vi "Gare ratio save FGV.vi"(7 "Command":T1(ring), 8 "error in (no error)":errorcluster, 10 "Gear Ratio":dbl=4.3, 11 "File Path":path) -> (0 "error out":errorcluster, 2 "Gear Ratio":dbl=4.3)   [LabVIEW 2018]
doc: "This Subvi usde for CSV Initialize ,Read, Write and close.\nIntilise case; we check File avaliblity in not found create csv file\nRead Case ; Read data from csv file"
uses:
  <vilib>/Utility/file.llb/Write Delimited Spreadsheet (string).vi
  <vilib>/Utility/file.llb/Read Delimited Spreadsheet (string).vi
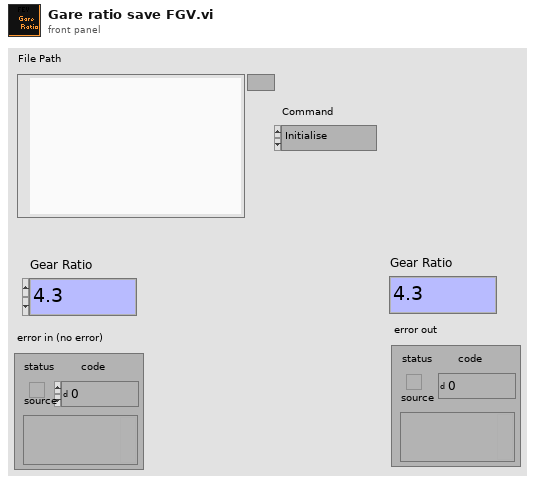
[diagram p1: front panel]
types:
  T1 = enum16{"Initialise", "Read Data", "Write Data", "Close"}
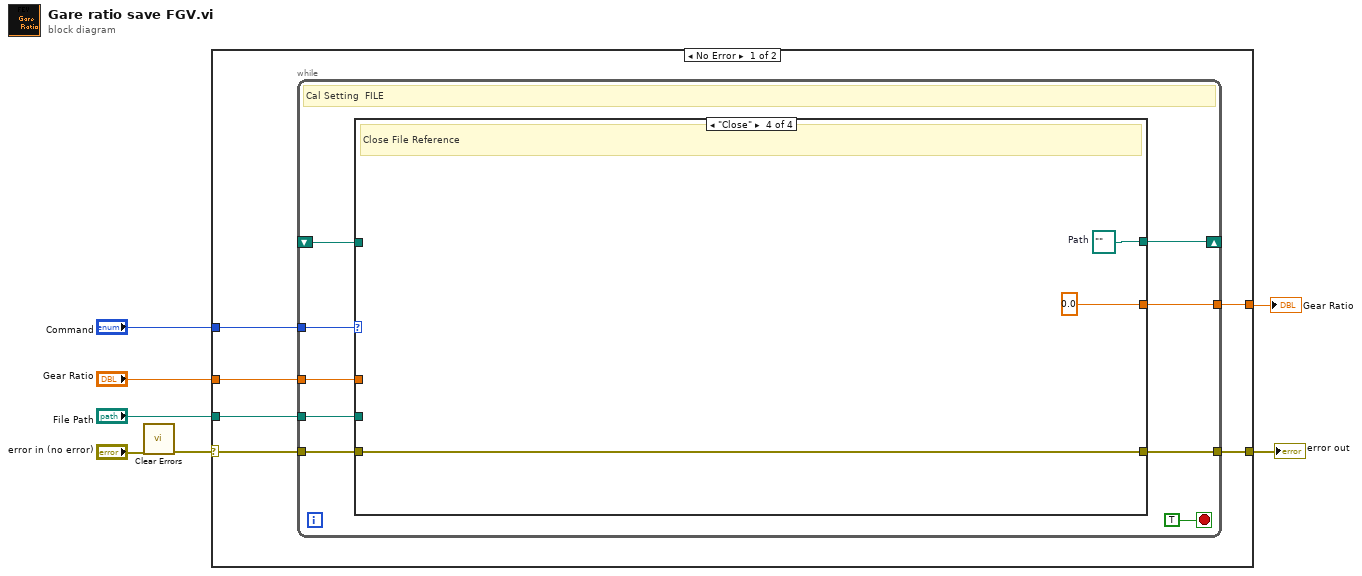
[diagram p0: block diagram]
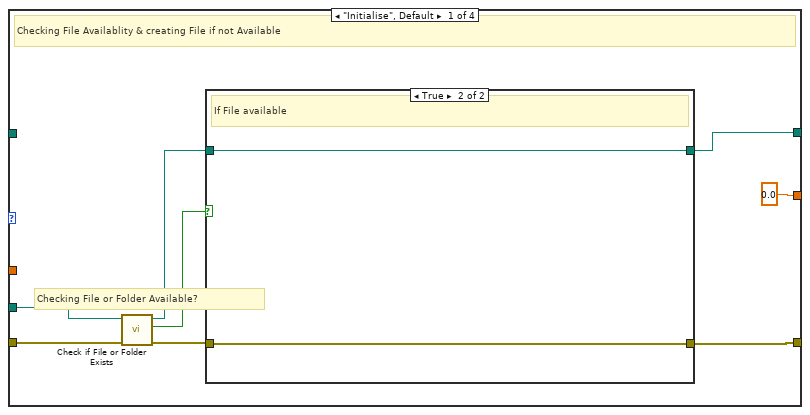
[diagram p2: hidden frame]
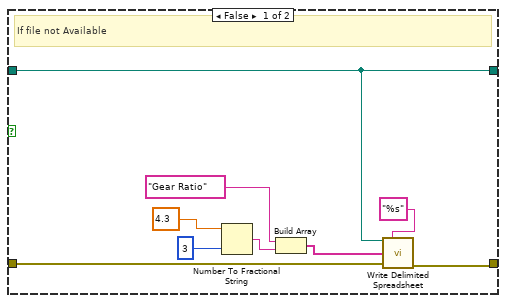
[diagram p3: hidden frame]
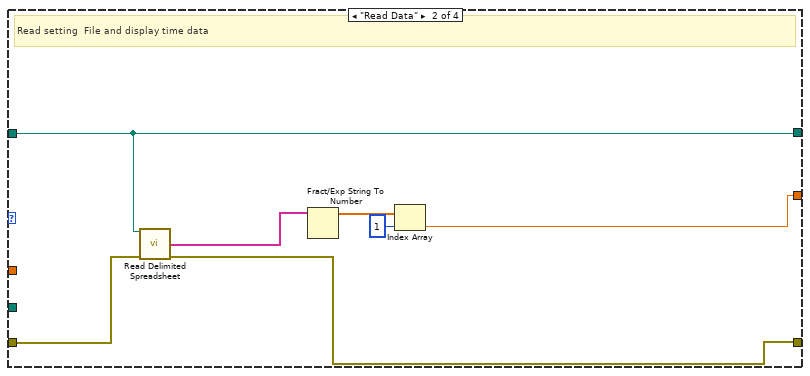
[diagram p4: hidden frame]
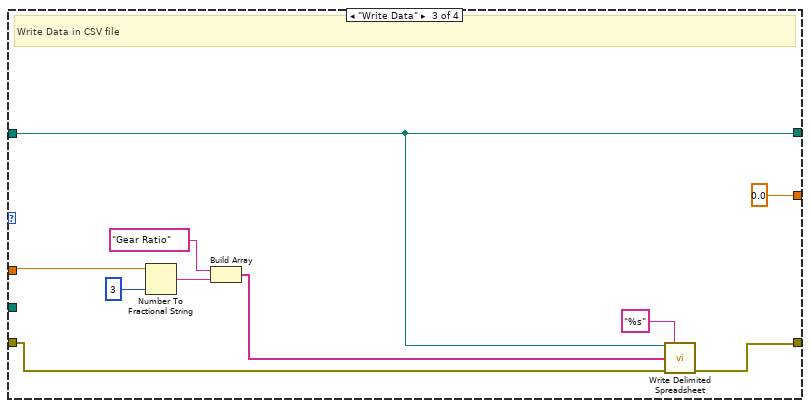
[diagram p5: hidden frame]
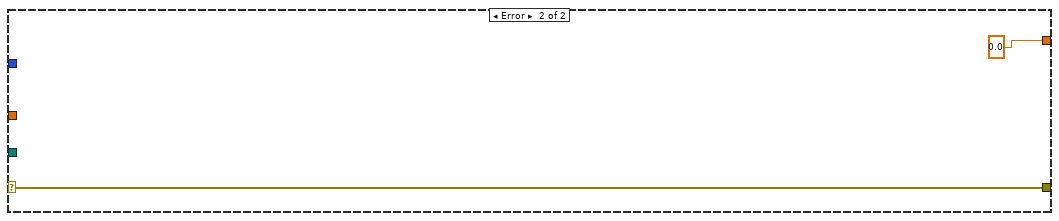
[diagram p6: hidden frame]
diagram:
  n1 = call <vilib>:"Clear Errors.vi"("error in (no error)"="error in (no error)") -> ("error out"=w3:errorcluster)  [unwired: 5 in, 1 out]
  n2 = case shown="No Error" w3 {
    selector: w3 -> [w12 w63]
    tunnel: [w11 w63] -> w6
    tunnel: "Command" -> [w13 _]
    tunnel: "File Path" -> [w10 _]
    tunnel: [w9 0.0 ("Gear Ratio")] -> w2
    tunnel: "Gear Ratio" -> [w8 _]
    frame No Error {
      n3 = while {
        shift-right: [w17] -> _
        shift-left: _ -> [w16]
        tunnel: w13 -> [w21]
        tunnel: w12 -> [w20]
        tunnel: [w19] -> w11
        tunnel: w10 -> [w18]
        tunnel: [w15] -> w9
        tunnel: w8 -> [w14]
        stop <- TRUE stop-if-true
        # "Cal Setting  FILE"
        n4 = case shown="\"Close\"" w21 {
          tunnel: w20 -> [w30 w47 w55 w61]
          tunnel: [w24 w46 w54 w61] -> w19
          tunnel: w18 -> [w29 _ _ _]
          tunnel: [w27 w48 w53 w60] -> w17
          tunnel: w16 -> [_ w48 w53 _]
          tunnel: [0.0 ("Gear Ratio") w43 0.0 ("Gear Ratio") 0.0 ("Gear Ratio")] -> w15
          tunnel: w14 -> [_ _ w51 _]
          frame "Initialise", Default {
            # "Checking File or Folder Available?"
            # "Checking File Availablity & creating File if not Available"
            n5 = call <vilib>:"Check if File or Folder Exists.vi"("error in (no error)"=w30, "path"=w29) -> ("error out"=w25:errorcluster, "file or folder exists?"=w28:bool, "dup path"=w26:path)  [unwired: 7 in]
            n6 = case shown="True" w28 {
              tunnel: [w37 w41] -> w27
              tunnel: w26 -> [w37 w41]
              tunnel: w25 -> [w35 w40]
              tunnel: [w34 w40] -> w24
              frame False {
                # "If file not Available"
                n7 = Number To Fractional String(number=4.3, precision (6)=i16 3) -> (F-format string=w39:string)  [unwired: 2 in]
                n8 = Build Array("Gear Ratio" ("Output Load Offset (Kg)"), w39) -> (w31:string[])
                n9 = call-poly <vilib>:"Write Delimited Spreadsheet.vi"("file path (dialog if empty)"=w37, "format (%s)"="%s", "1D data"=w31, "error in (no error)"=w35) -> ("error out"=w34:errorcluster)  [unwired: 10 in, 1 out]
              }
              frame True {
                # "If File available"
              }
            }
          }
          frame "Read Data" {
            # "Read setting  File and display time data"
            n10 = call-poly <vilib>:"Read Delimited Spreadsheet.vi"("file path (dialog if empty)"=w48, "error in (no error)"=w47) -> ("first row"=w44:string[], "error out"=w46:errorcluster)  [unwired: 8 in, 4 out]
            n11 = Fract/Exp String To Number(string=w44) -> (number=w45:dbl[])  [unwired: 3 in, 1 out]
            n12 = Index Array(array=w45, index=1) -> (element=w43:dbl)
          }
          frame "Write Data" {
            # "Write Data in CSV file"
            n13 = Number To Fractional String(number=w51, precision (6)=i16 3) -> (F-format string=w58:string)  [unwired: 2 in]
            n14 = Build Array("Gear Ratio" ("Output Load Offset (Kg)"), w58) -> (w49:string[])
            n15 = call-poly <vilib>:"Write Delimited Spreadsheet.vi"("file path (dialog if empty)"=w53, "format (%s)"="%s", "1D data"=w49, "error in (no error)"=w55) -> ("error out"=w54:errorcluster)  [unwired: 10 in, 1 out]
          }
          frame "Close" {
            w60 = path ""  # Path
            # "Close File Reference"
          }
        }
      }
    }
    frame Error {
    }
  }
  "error out" <- w6
  "Gear Ratio" <- w2
